vi "svm_cross_validation.vi"(8 "error in (no error)":errorcluster, 9 "Nr fold":i32 caption="Nr fold (LOO)", 10 "Parameters":T1, 11 "Problem":T4) -> (0 "error out":errorcluster, 3 "Target":dbl[](array[numeric]) caption="Target (Predicted labels)")   [LabVIEW 2015]
uses:
  Controls/svm_problem.ctl
  Controls/svm_node.ctl
  Controls/svm_parameter.ctl
  Controls/svm_type.ctl
  Controls/svm_kernel_type.ctl
  bin/x64/LabVIEW-libsvm.dll
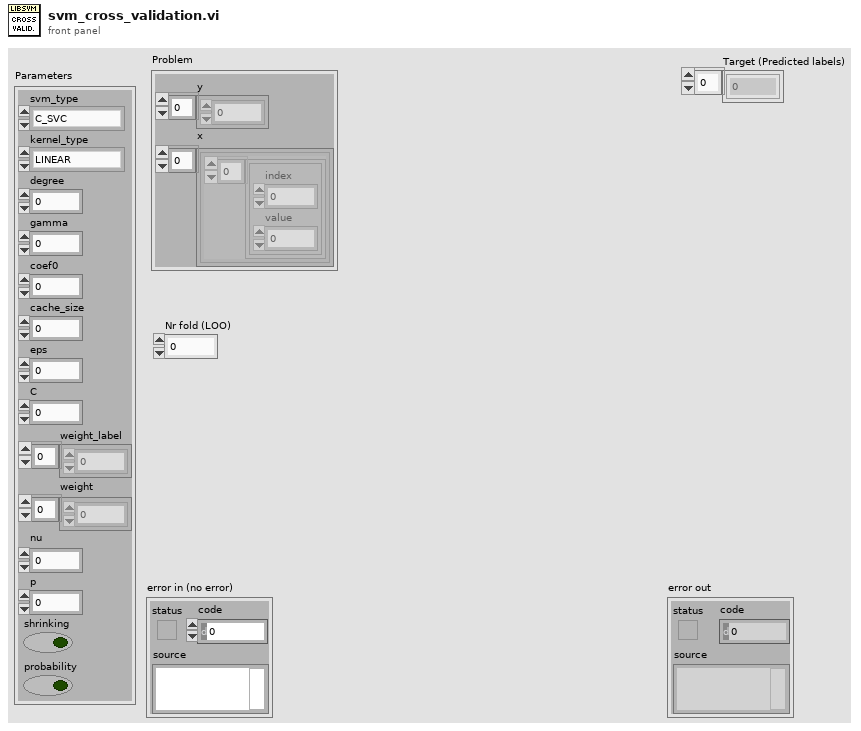
[diagram p1: front panel]
types:
  T1 = typedef "svm_parameter.ctl" = cluster{"svm_type":T2, "kernel_type":T3, "degree":i32, "gamma":dbl, "coef0":dbl, "cache_size":dbl, "eps":dbl, "C":dbl, "weight_label":i32[], "weight":dbl[], "nu":dbl, "p":dbl, "shrinking":bool, "probability":bool}
  T2 = typedef "svm_type.ctl" = enum32{"C_SVC", "NU_SVC", "ONE_CLASS", "EPSILON_SVR", "NU_SVR"}
  T3 = typedef "svm_kernel_type.ctl" = enum32{"LINEAR", "POLY", "RBF", "SIGMOID", "PRECOMPUTED"}
  T4 = typedef "svm_problem.ctl" = cluster{"y":dbl[], "x":cluster{T5[]}[]}
  T5 = typedef "svm_node.ctl" = cluster{"index":i32, "value":dbl}
  T6 = typedef "svm_problem_padded.ctl" = cluster{"y":dbl[], "x":cluster{T7[]}[]}
  T7 = typedef "svm_node_padded.ctl" = cluster{"index":i32, "padding":i32, "value":dbl}
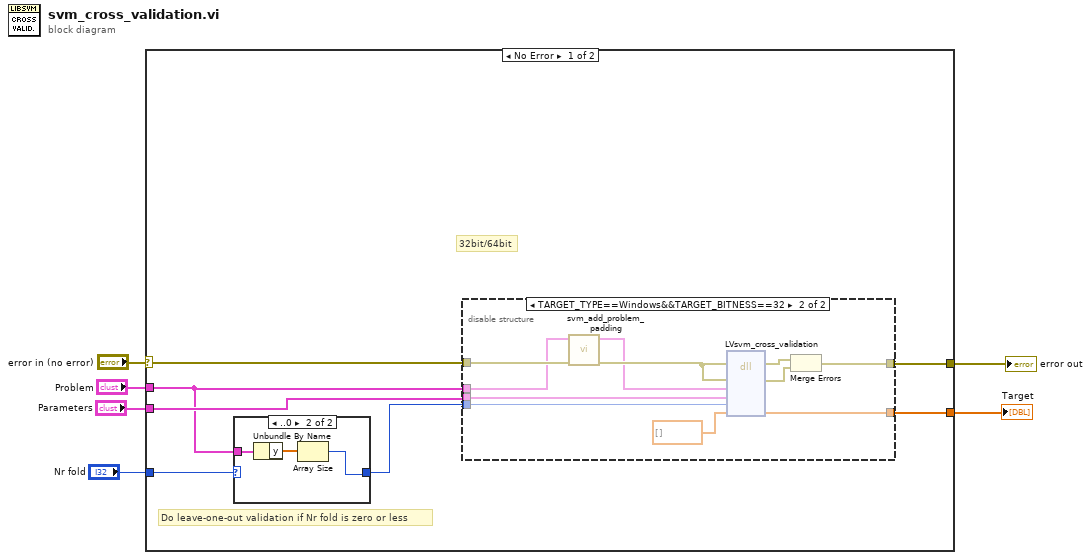
[diagram p0: block diagram]
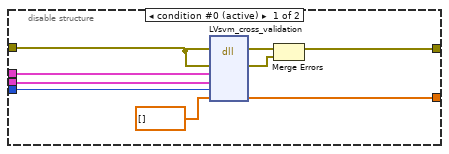
[diagram p2: hidden frame]
diagram:
  n1 = case shown="No Error" "error in (no error)" {
    selector: "error in (no error)" -> [w13 w38]
    tunnel: [w12 w38] -> w5
    tunnel: "Nr fold" -> [w9 _]
    tunnel: "Problem" -> [w8 _]
    tunnel: "Parameters" -> [w11 _]
    tunnel: [w10 _] -> w1
    frame No Error {
      # "32bit/64bit"
      # "Do leave-one-out validation if Nr fold is zero or less"
      n2 = case shown="..0" w9 {
        selector: w9 -> [w34 _]
        tunnel: w8 -> [_ w37]
        tunnel: [w34 w35] -> w7
        frame Default {
        }
        frame ..0 {
          n3 = Unbundle By Name(w37) -> ("y"=w36:dbl[])
          n4 = Array Size(array=w36) -> (size(s)=w35:i32)
        }
      }
      n5 = disable-structure shown="TARGET_TYPE==Windows&&TARGET_BITNESS==32" {
        disable-tunnel: [w19 w30] -> w12
        disable-tunnel: [w15 w29] -> w10
        disable-tunnel: w11 -> [w16 w28]
        disable-tunnel: w7 -> [w14 w27]
        disable-tunnel: w13 -> [w18 w26]
        disable-tunnel: w8 -> [w17 w24]
        frame condition #0 (active) {
          n6 = dll-call lib="C:/dev/LabVIEW-libsvm/LabVIEW/bin/x64/LabVIEW-libsvm.dll" fn="LVsvm_cross_validation"(error in=w18, "lvErr"=w18, "prob_in"=w17, "param_in"=w16, "nr_fold"=w14, "target_out"=dbl[] []) -> (error out=w22:errorcluster, "lvErr"=w21:errorcluster, "target_out"=w15:dbl[])  [unwired: 6 in, 1 out]
          n7 = Merge Errors(w22, w21) -> (w19:errorcluster)
        }
        frame condition #1 {
          n8 = call "svm_add_problem_padding.vi"("error in (no error)"=w26, "problem"=w24) -> ("error out"=w25:errorcluster, "padded problem"=w23:T6)  [unwired: 8 in]
          n9 = dll-call lib="C:/dev/LabVIEW-libsvm/LabVIEW/bin/x64/LabVIEW-libsvm.dll" fn="LVsvm_cross_validation"(error in=w25, "lvErr"=w25, "prob_in"=w23, "param_in"=w28, "nr_fold"=w27, "target_out"=dbl[] []) -> (error out=w33:errorcluster, "lvErr"=w32:errorcluster, "target_out"=w29:dbl[])  [unwired: 6 in, 1 out]
          n10 = Merge Errors(w33, w32) -> (w30:errorcluster)
        }
      }
    }
    frame Error {
    }
  }
  "error out" <- w5
  "Target" <- w1
